vi "Launcher.vi"() -> ()   [LabVIEW 2014, in "POLARIS Target Focus Actor.lvlib"]
uses:
  POLARIS Target Focus Actor.lvlib
  <vilib>/userdefined/High Color/IMAQdx.ctl
  Utility/Width Method.ctl
  POLARIS Target Focus Actor/POLARIS Target Focus Actor.lvclass
  POLARIS Target Focus Actor/POLARIS Target Focus Actor.lvclass/POLARIS Target Focus Actor.ctl
  <vilib>/ActorFramework/Message Enqueuer/Message Enqueuer.lvclass/Message Enqueuer.ctl
  POLARIS Target Focus Actor/Write Method.vi
  <vilib>/ActorFramework/Message Enqueuer/Enqueue.vi
  <vilib>/Utility/config.llb/Read Key (Path).vi
  <vilib>/Utility/config.llb/Read Key (U32).vi
  <vilib>/Utility/config.llb/Read Key (String).vi
  Applications/HIJ Vision Camera App/HIJ Vision Camera App/Write Start Camera.vi
  Applications/HIJ Vision Camera App/HIJ Vision Camera App/Write my ConfigDir.vi
  Applications/HIJ Vision Camera App/HIJ Vision Camera App/Write my WorkDir.vi
  <vilib>/ActorFramework/Message Priority Queue/Priority Enqueue.vi
  <vilib>/Utility/config.llb/Write Key (Path).vi
  <vilib>/Utility/config.llb/Write Key (I32).vi
  <vilib>/Utility/config.llb/Write Key (String).vi
  Shared Code/Viewable Actor/ViewableActor Messages/Open Front Panel Msg/Open Front Panel Msg.lvclass
  <vilib>/ActorFramework/Actor/Actor.lvclass
  <vilib>/Utility/config.llb/NI_LVConfig.lvlib
  Utility/POLARIS Vision utility.lvlib
panel:
  in  "Method":T1
  in  "UI Cnfg":path
  in  "CLine Parameter":string
  in  "Focus Camera":T2="TestCam"
  out "error out":errorcluster
  in  "Start ConfigDir":path=path "C:/Users/user/Desktop/test/ConfigDir"
  in  "Start WorkDir":path=path "C:/Users/user/Desktop/test/WorkDir"
  in  "RUN_STOP":bool
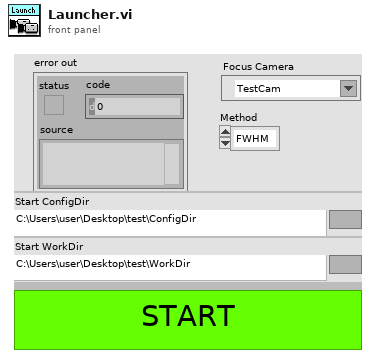
[diagram p1: front panel]
types:
  T1 = typedef "POLARIS Vision utility.lvlib/Width Method.ctl" = enum16{"FWHM", "1/e", "1/e^2", "80%", "90%"}
  T2 = typedef "IMAQdx.ctl" = refnum<k21>
  T3 = typedef "NI_LVConfig.lvlib/Config Data RefNum.ctl" = refnum<k1>
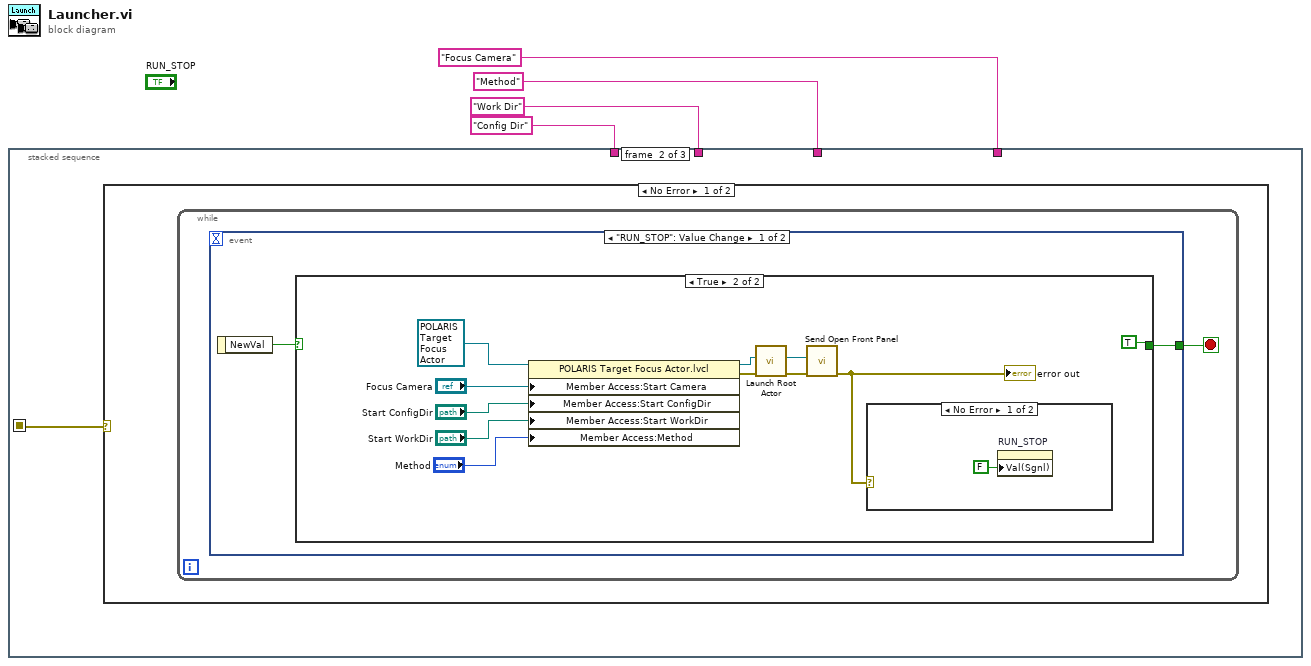
[diagram p0: block diagram]
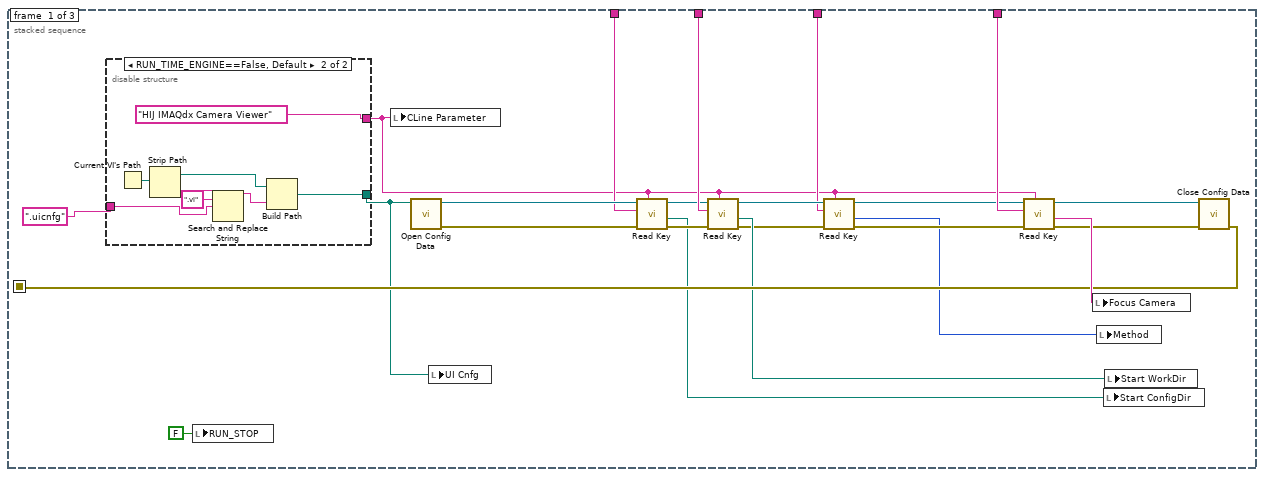
[diagram p2: hidden frame]
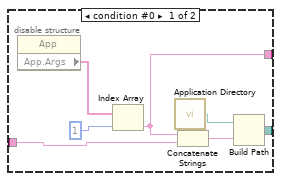
[diagram p3: hidden frame]
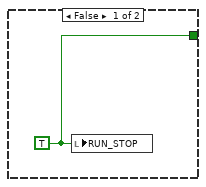
[diagram p4: hidden frame]
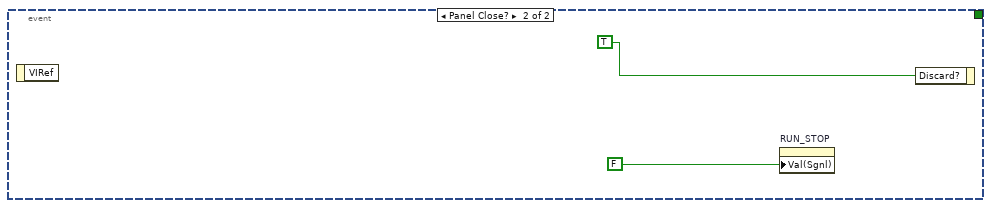
[diagram p6: hidden frame]
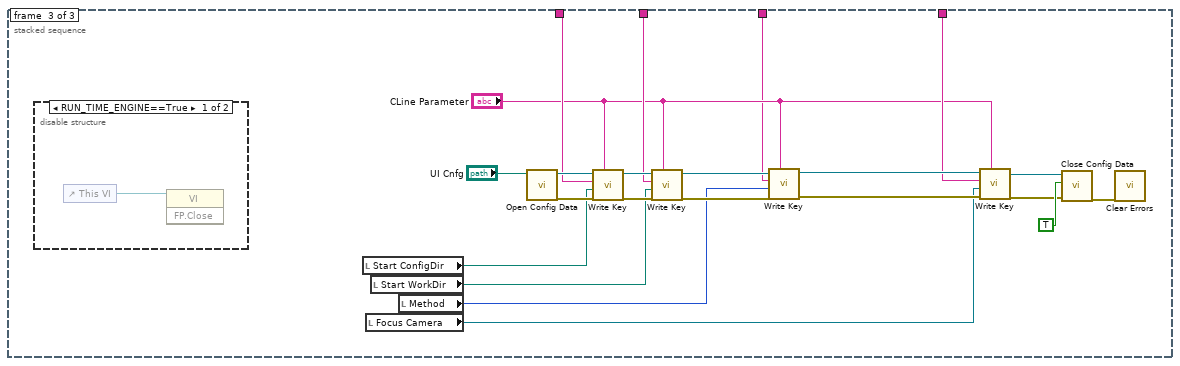
[diagram p8: hidden frame]
diagram:
  n1 = stacked-sequence {
    seq-local: [w22 _ _] -> [_ w43 _]
    tunnel: "Config Dir" ("key") -> [w23 _ w80]
    tunnel: "Work Dir" ("key") -> [w20 _ w69]
    tunnel: "Focus Camera" ("key") -> [w19 _ w68]
    tunnel: "Method" ("key") -> [w7 _ w62]
    frame #0 {
      n2 = disable-structure shown="RUN_TIME_ENGINE==False, Default" {
        disable-tunnel: [w30 w36] -> w21
        disable-tunnel: ".uicnfg" ("string") -> [w29 w39]
        disable-tunnel: [w28 "HIJ IMAQdx Camera Viewer"] -> w6
        frame condition #0 {
          n3 = property class="App"() -> ("App.Args"=w34:string[])  [unwired: 2 in, 2 out]
          n4 = Index Array(array=w34, index=1) -> (element=w28:string)
          n5 = call <vilib>:"Application Directory.vi"() -> ("Application Directory"=w32:path)
          n6 = Concatenate Strings(w28, w29) -> (w31:string)
          n7 = Build Path(base path=w32, name or relative path=w31) -> (appended path=w30:path)
        }
        frame condition #1 (active) {
          n8 = Current VI's Path() -> (path=w42:path)
          n9 = Strip Path(path=w42) -> (stripped path=w37:path, name=w41:string)
          n10 = Search and Replace String(input string=w41, search string=".vi", replace string=w39) -> (result string=w38:string)  [unwired: 5 in, 3 out]
          n11 = Build Path(base path=w37, name or relative path=w38) -> (appended path=w36:path)
        }
      }
      n12 = local write "RUN_STOP"(FALSE ("RUN_STOP")) -> ()
      n13 = local write "CLine Parameter"(w6) -> ()
      n14 = call <vilib>:"Open Config Data.vi"("configuration file path"=w21) -> ("error out"=w25:errorcluster, "refnum"=w24:T3)  [unwired: 8 in, 1 out]
      n15 = local write "UI Cnfg"(w21) -> ()
      n16 = call-poly <vilib>:"Read Key.vi"("section"=w6, "error in (no error)"=w25, "key"=w23, "refnum"=w24) -> ("error out"=w17:errorcluster, "value"=w13:path, "refnum out"=w18:T3)  [unwired: 4 in, 1 out]
      n17 = call-poly <vilib>:"Read Key.vi"("section"=w6, "error in (no error)"=w17, "key"=w20, "refnum"=w18) -> ("error out"=w9:errorcluster, "value"=w12:path, "refnum out"=w11:T3)  [unwired: 4 in, 1 out]
      n18 = call-poly <vilib>:"Read Key.vi"("section"=w6, "error in (no error)"=w9, "key"=w7, "refnum"=w11) -> ("error out"=w8:errorcluster, "value"=w5:u32, "refnum out"=w10:T3)  [unwired: 4 in, 1 out]
      n19 = call-poly <vilib>:"Read Key.vi"("section"=w6, "error in (no error)"=w8, "key"=w19, "refnum"=w10) -> ("error out"=w15:errorcluster, "value"=w27:string, "refnum out"=w16:T3)  [unwired: 4 in, 1 out]
      n20 = local write "Focus Camera"(w27) -> ()
      n21 = local write "Method"(w5) -> ()
      n22 = local write "Start ConfigDir"(w13) -> ()
      n23 = local write "Start WorkDir"(w12) -> ()
      n24 = call <vilib>:"Close Config Data.vi"("error in (no error)"=w15, "refnum"=w16) -> ("error out"=w22:errorcluster)  [unwired: 8 in, 1 out]
    }
    frame #1 {
      n25 = case shown="No Error" w43 {
        frame No Error {
          n26 = while {
            stop <- w44 stop-if-true
            n27 = event shown="[0] \"RUN_STOP\": Value Change" {
              selector: _ -> [_ _]
              dyn-events: _ -> [_ _]
              timeout: _ -> [_ _]
              tunnel: [w46 _] -> w44
              event "RUN_STOP": Value Change {
                n28 = event-data() -> ("NewVal"=w45:bool)  [unwired: 1 in]
                n29 = case shown="True" w45 {
                  tunnel: [w47 TRUE] -> w46
                  frame False {
                    w47 = TRUE ("RUN_STOP")
                    n30 = local write "RUN_STOP"(w47) -> ()
                  }
                  frame True {
                    n31 = property class="POLARIS Target Focus Actor.lvcl"(reference=refnum<class "POLARIS Target Focus Actor.lvclass"> refnum ("POLARIS Target Focus Actor.lvlib:POLARIS Target Focus Actor.lvclass"), "Member Access:Start Camera"="Focus Camera", "Member Access:Start ConfigDir"="Start ConfigDir", "Member Access:Start WorkDir"="Start WorkDir", "Member Access:Method"="Method") -> (reference out=w53:refnum<class "POLARIS Target Focus Actor.lvclass">, error out=w54:errorcluster)  [unwired: 1 in]
                    n32 = call <vilib>:"Launch Root Actor.vi"("error in (no error)"=w54, "Actor"=w53) -> ("error out"=w51:errorcluster, "Actor's Enqueuer"=w52:refnum<class "Message Enqueuer.lvclass">)  [unwired: 8 in]
                    n33 = call "Send Open Front Panel.vi"("error in (no error)"=w51, "Message Enqueuer"=w52) -> ("error out"=w50:errorcluster)  [unwired: 8 in, 1 out]
                    "error out" <- w50
                    n34 = case shown="No Error" w50 {
                      frame No Error {
                        n35 = property on="RUN_STOP" class="Bool (strict)"("Val(Sgnl)"=FALSE ("Value (Signaling)")) -> ()  [unwired: 2 in, 2 out]
                      }
                      frame Error {
                      }
                    }
                  }
                }
              }
              event Panel Close? {
                n36 = event-data() -> ()  [unwired: 1 in, 1 out]
                n37 = property on="RUN_STOP" class="Bool (strict)"("Val(Sgnl)"=FALSE ("Value (Signaling)")) -> ()  [unwired: 2 in, 2 out]
                n38 = event-data("Discard?"=TRUE) -> ()  [unwired: 1 in, 1 out]
              }
            }
          }
        }
        frame Error {
        }
      }
    }
    frame #2 {
      n39 = disable-structure shown="RUN_TIME_ENGINE==True" {
        frame condition #0 {
          n40 = control-ref of="This VI"() -> (w84:refnum<vi>)
          n41 = invoke class="VI" method="FP.Close"(reference=w84) -> ()  [unwired: 2 in, 3 out]
        }
        frame condition #1 (active) {
        }
      }
      n42 = local read "Start ConfigDir"() -> (w71:path)
      n43 = local read "Focus Camera"() -> (w66:T2)
      n44 = local read "Start WorkDir"() -> (w70:path)
      n45 = local read "Method"() -> (w63:T1)
      n46 = call <vilib>:"Open Config Data.vi"("configuration file path"="UI Cnfg") -> ("error out"=w79:errorcluster, "refnum"=w82:T3)  [unwired: 8 in, 1 out]
      n47 = call-poly <vilib>:"Write Key.vi"("section"="CLine Parameter", "error in (no error)"=w79, "value"=w71, "key"=w80, "refnum"=w82) -> ("error out"=w78:errorcluster, "refnum out"=w83:T3)  [unwired: 4 in, 1 out]
      n48 = call-poly <vilib>:"Write Key.vi"("section"="CLine Parameter", "error in (no error)"=w78, "value"=w70, "key"=w69, "refnum"=w83) -> ("error out"=w74:errorcluster, "refnum out"=w75:T3)  [unwired: 4 in, 1 out]
      n49 = call-poly <vilib>:"Write Key.vi"("section"="CLine Parameter", "error in (no error)"=w74, "value"=w63, "key"=w62, "refnum"=w75) -> ("error out"=w73:errorcluster, "refnum out"=w72:T3)  [unwired: 4 in, 1 out]
      n50 = call-poly <vilib>:"Write Key.vi"("section"="CLine Parameter", "error in (no error)"=w73, "value"=w66, "key"=w68, "refnum"=w72) -> ("error out"=w65:errorcluster, "refnum out"=w64:T3)  [unwired: 4 in, 1 out]
      n51 = call <vilib>:"Close Config Data.vi"("error in (no error)"=w65, "write file if changed (T)"=TRUE, "refnum"=w64) -> ("error out"=w77:errorcluster)  [unwired: 7 in, 1 out]
      n52 = call <vilib>:"Clear Errors.vi"("error in (no error)"=w77) -> ()  [unwired: 5 in, 2 out]
    }
  }
